vi "Acquire Until Falling Edge.vi"() -> ()   [LabVIEW 2017]
uses:
  controls/User Specified Data.ctl
  controls/HW Configuration.ctl
  controls/Analysis Configuration.ctl
  controls/New Data Behavior.ctl
  controls/Signal Configuration.ctl
  <vilib>/Utility/error.llb/DialogType.ctl
  <vilib>/DAQmx/read.llb/DAQmx Read (Analog 1D Wfm NChan NSamp).vi
  <vilib>/DAQmx/create/channels.llb/DAQmx Create Channel (AI-Voltage-Basic).vi
  <vilib>/DAQmx/configure/timing.llb/DAQmx Timing (Sample Clock).vi
  <vilib>/DAQmx/configure/trigger.llb/DAQmx Start Trigger (Digital Edge).vi
  <vilib>/DAQmx/configure/trigger.llb/DAQmx Reference Trigger (Digital Edge).vi
  <vilib>/DAQmx/miscellaneous.llb/DAQmx Fill In Error Info.vi
  <resource>/objmgr/daqmx.rc
panel:
  in  "Buffer Size":u32=100000
  out "data":waveform(dbl)[](array[waveform])
  in  "Post-Trigger Samples":u32
  in  "Samples Per Read":u32=100
  in  "User Specified":T1={"Hardware Configuration"={"Signal Channel"="PXI1Slot7/ao0", "Response Channel"="PXI1Slot7/ai0", "Trigger Channel"="/PXI1Slot7/PFI0", "Number of acquisitions"=0.0}, "Analysis Configuration"={"Statistics"=TRUE}, "Signal Type"=enum."Single Chirp", "New Data Behavior"=enum."Replace", "Signal Configuration"={"Chirp Amplitude"=0.1, "I/O Limit"=10.0, "Sample Rate"=1000000.0, "Chirp Duration (s)"=10000000.0, "Upper Frequency"=0.0, "Lower Frequency"=0.0, "Windowing"=enum."None"}}
  out "Waveform Graph":waveform(dbl)[](graph)
  in  "error in":errorcluster
  out "error out":errorcluster
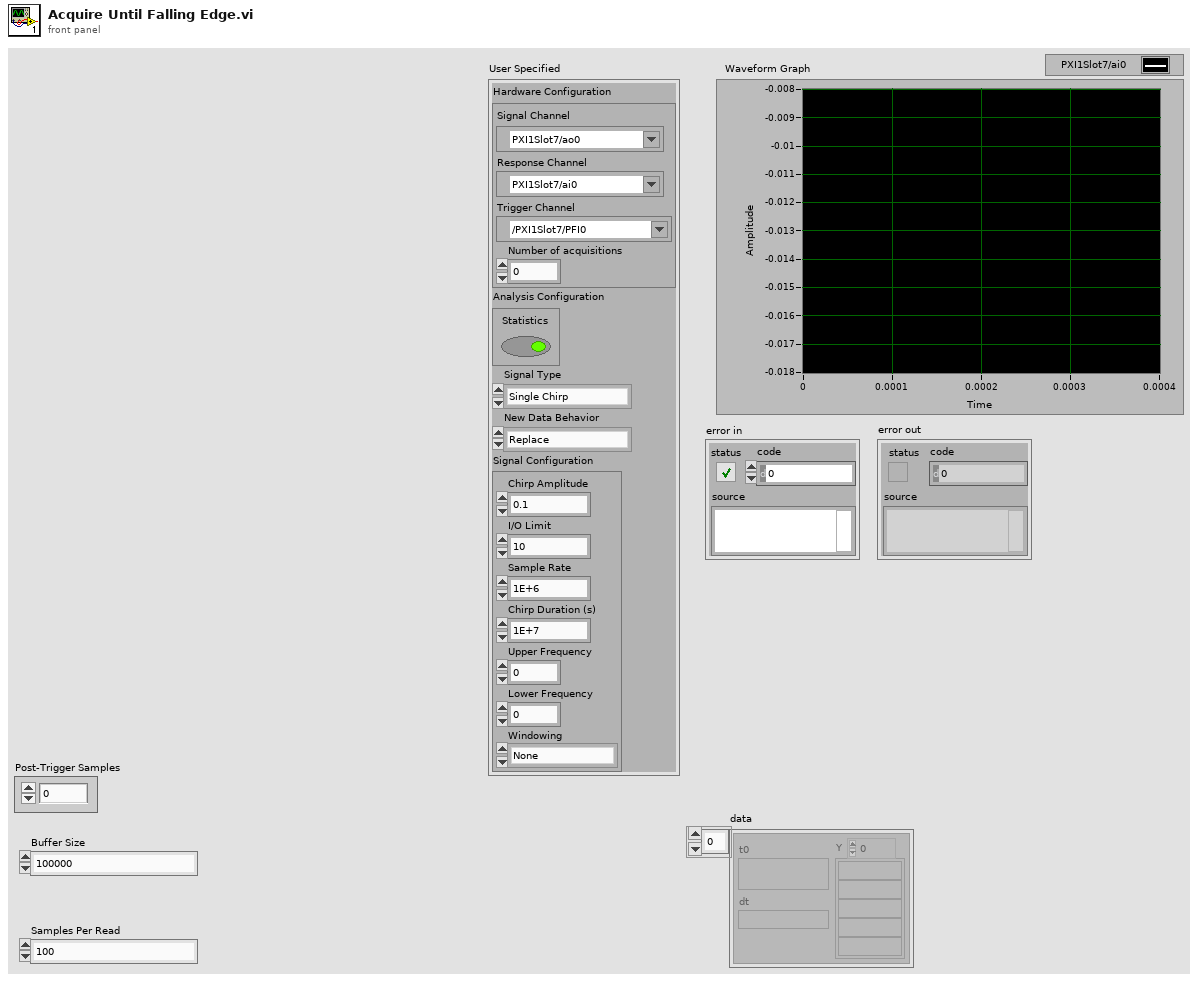
[diagram p1: front panel]
types:
  T1 = typedef "User Specified Data.ctl" = cluster{"Hardware Configuration":T2, "Analysis Configuration":T3, "Signal Type":enum16{"Single Chirp", "From Excel"}, "New Data Behavior":T4, "Signal Configuration":T5}
  T2 = typedef "HW Configuration.ctl" = cluster{"Signal Channel":tag, "Response Channel":tag, "Trigger Channel":tag, "Number of acquisitions":dbl}
  T3 = typedef "Analysis Configuration.ctl" = cluster{"Statistics":bool}
  T4 = typedef "New Data Behavior.ctl" = enum16{"Replace", "Overlay", "Append"}
  T5 = typedef "Signal Configuration.ctl" = cluster{"Chirp Amplitude":dbl, "I/O Limit":dbl, "Sample Rate":dbl, "Chirp Duration (s)":dbl, "Upper Frequency":dbl, "Lower Frequency":dbl, "Windowing":enum16{"None", "Exponential", "Flat top", "Hamming", "Hanning", "Kaiser-Bessel", "Rectangular"}}
  T6 = typedef "DialogType.ctl" = u16
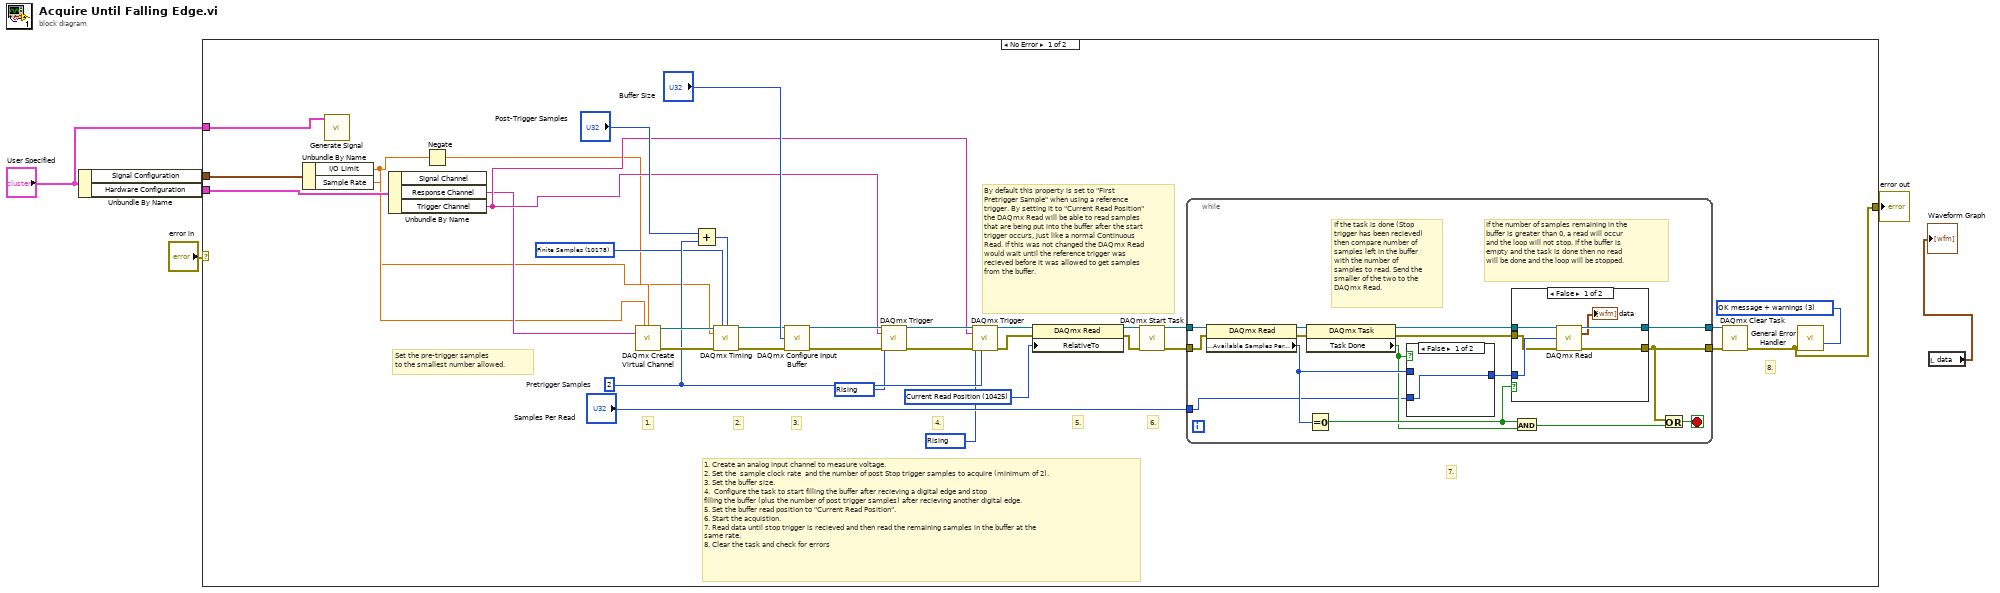
[diagram p0: block diagram]
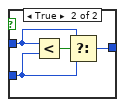
[diagram p3: hidden frame]
diagram:
  n1 = Unbundle By Name("User Specified") -> ("Signal Configuration"=w4:T5, "Hardware Configuration"=w3:T2)
  n2 = case shown="No Error" "error in" {
    selector: "error in" -> [_ w70]
    tunnel: w3 -> [w41 _]
    tunnel: [w9 w70] -> w6
    tunnel: w4 -> [w40 _]
    tunnel: "User Specified" -> [w39 _]
    frame No Error {
      w7 = 10280 items=["Rising"=10280, "Falling"=10171] ("edge")
      w8 = 10280 items=["Rising"=10280, "Falling"=10171] ("edge")
      w17 = 10425 items=["First Sample"=10424, "Current Read Position"=10425, "Reference Trigger"=10426, "First Pretrigger Sample"=10427, "Most Recent Sample"=10428] ("RelativeTo")
      w18 = u32 2  # Pretrigger Samples
      w15 = T6 3 items=["no dialog", "OK message", "continue or stop message", "OK message + warnings", "continue/stop + warnings"] ("type of dialog (OK msg:1)")
      w16 = 10178 items=["Finite Samples"=10178, "Continuous Samples"=10123] ("sample mode")
      # "Set the pre-trigger samples\nto the smallest number allowed."
      # "8."
      # "7."
      # "6."
      # "By default this property is set to \"First Pretrigger Sample\" when using a reference trigger. By setting it to \"Current Read Position\" the DAQmx Read will be able to read samples that are being put into the buffer after the start trigger occurs, just like a normal Continuous Read. If this was not changed the DAQmx Read would wait until the reference trigger was recieved before it was allowed to get samples from the buffer."
      # "5."
      # "1. Create an analog input channel to measure voltage.\n2. Set the  sample clock rate  and the number of post Stop trigger samples to acquire (minimum of 2).\n3. Set the buffer size.\n4.  Configure the task to start filling the buffer after recieving a digital edge and stop \nfilling the buffer (plus the number of post trigger samples) after recieving another digital edge.\n5. Set the buffer read position to \"Current Read Position\".\n6. Start the acquistion.\n7. Read data until stop trigger is recieved and then read the remaining samples in the buffer at the \nsame rate.\n8. Clear the task and check for errors"
      # "4."
      # "3."
      # "2."
      # "1."
      n3 = Unbundle By Name(w40) -> ("I/O Limit"=w11:dbl, "Sample Rate"=w10:dbl)
      n4 = call "Generate Signal.vi"("User Specified"=w39) -> ()  [unwired: 7 in, 4 out]
      n5 = Unbundle By Name(w41) -> ("Response Channel"=w13:tag, "Trigger Channel"=w14:tag)  [unwired: 1 out]
      n6 = Negate(x=w11) -> (-x=w12:dbl)
      n7 = call-poly <vilib>:"DAQmx Create Virtual Channel.vi"("maximum value"=w11, "minimum value"=w12, "physical channels"=w13) -> ("task out"=w21:refnum<k21>, "error out"=w19:errorcluster)  [unwired: 11 in]
      n8 = Add(x="Post-Trigger Samples", y=w18) -> (x+y=w36:u32)
      n9 = call-poly <vilib>:"DAQmx Timing.vi"("task/channels in"=w21, "sample mode"=w16, "samples per channel"=w36, "rate"=w10, "error in"=w19) -> ("task out"=w24:refnum<k21>, "error out"=w25:errorcluster)  [unwired: 9 in]
      n10 = call <vilib>:"DAQmx Configure Input Buffer.vi"("task/channels in"=w24, "buffer size (in samples per channel)"="Buffer Size", "error in"=w25) -> ("task out"=w32:refnum<k21>, "error out"=w33:errorcluster)  [unwired: 11 in]
      n11 = call-poly <vilib>:"DAQmx Trigger.vi"("task/channels in"=w32, "source"=w14, "edge"=w8, "error in"=w33) -> ("task out"=w35:refnum<k21>, "error out"=w34:errorcluster)  [unwired: 10 in]
      n12 = call-poly <vilib>:"DAQmx Trigger.vi"("task/channels in"=w35, "source"=w14, "edge"=w7, "error in"=w34, "pretrigger samples per channel"=w18) -> ("task out"=w27:refnum<k21>, "error out"=w28:errorcluster)  [unwired: 9 in]
      n13 = property class="DAQmx Read"(reference=w27, error in=w28, "RelativeTo"=w17) -> (reference out=w30:refnum<k21>, error out=w29:errorcluster)
      n14 = call <vilib>:"DAQmx Start Task.vi"("task/channels in"=w30, "error in"=w29) -> ("task out"=w22:refnum<k21>, "error out"=w20:errorcluster)  [unwired: 12 in]
      n15 = while {
        tunnel: w20 -> [w54]
        tunnel: [w43] -> w31
        tunnel: w22 -> [w55]
        tunnel: [w53] -> w23
        tunnel: "Samples Per Read" -> [w42]
        stop <- w56 stop-if-true
        # "If the number of samples remaining in the\nbuffer is greater than 0, a read will occur\nand the loop will not stop. If the buffer is \nempty and the task is done then no read \nwill be done and the loop will be stopped."
        # "If the task is done (Stop trigger has been recieved) then compare number of samples left in the buffer\nwith the number of samples to read. Send the smaller of the two to the DAQmx Read."
        n16 = property class="DAQmx Read"(reference=w55, error in=w54) -> (reference out=w51:refnum<k21>, error out=w50:errorcluster, "Status:Available Samples Per Channel"=w52:u32)
        n17 = property class="DAQmx Task"(reference=w51, error in=w50) -> (reference out=w47:refnum<k21>, error out=w48:errorcluster, "Task Done"=w45:bool)
        n18 = Equal To 0?(x=w52) -> (x = 0?=w46:bool)
        n19 = case shown="False" w45 {
          tunnel: w52 -> [_ w68]
          tunnel: w42 -> [w65 w67]
          tunnel: [w65 w66] -> w49
          frame False {
          }
          frame True {
            n20 = Less?(x=w68, y=w67) -> (x < y?=w69:bool)
            n21 = Select(t=w68, s=w69, f=w67) -> (s? t:f=w66:u32)
          }
        }
        n22 = case shown="False" w46 {
          tunnel: [w62 w64] -> w43
          tunnel: [w61 w63] -> w53
          tunnel: w49 -> [w60 _]
          tunnel: w48 -> [w59 w64]
          tunnel: w47 -> [w58 w63]
          frame False {
            n23 = call-poly <vilib>:"DAQmx Read.vi"("task/channels in"=w58, "number of samples per channel"=w60, "error in"=w59) -> ("task out"=w61:refnum<k21>, "data"=→"data":waveform(dbl)[], "error out"=w62:errorcluster)  [unwired: 10 in]
          }
          frame True {
          }
        }
        n24 = And(x=w46, y=w45) -> (x .and. y?=w44:bool)
        n25 = Or(x=w43, y=w44) -> (x .or. y?=w56:bool)
      }
      n26 = call <vilib>:"DAQmx Clear Task.vi"("task in"=w23, "error in"=w31) -> ("error out"=w9:errorcluster)  [unwired: 13 in]
      n27 = call <vilib>:"General Error Handler.vi"("type of dialog (OK msg:1)"=w15, "error in (no error)"=w9) -> ()  [unwired: 9 in, 5 out]
    }
    frame Error {
    }
  }
  "error out" <- w6
  n28 = local read "data"() -> (→"Waveform Graph":waveform(dbl)[])
